vi "Main.vi"() -> ()   [LabVIEW 2017, in "Server.lvlib"]
doc: "This is the Main VI of the Dashboard Server Application. It consists of a QMH with several Loops. See the loop descriptions for details."
uses:
  Server.lvlib
  TypeDefs/SR List.ctl
  TypeDefs/SR Data.ctl
  TypeDefs/ClientList.ctl
  TypeDefs/ClientData.ctl
  SubLibs/Message Queue/EnqueueMessage(Single).vi
  <vilib>/Utility/error.llb/Error Cluster From Error Code.vi
  <vilib>/ErrorRing/Error Ring.xnode
  SubLibs/Message Queue/Message Queue.lvlib
  SubLibs/ErrorLogger/ErrorLogger.lvlib
  SubLibs/Oracle/Oracle.lvlib
  SubLibs/WebServiceCommunication/WebServiceCommunication.lvlib
  SubLibs/Logging/Logging.lvlib
  SubLibs/Timing/Timing.lvlib
  SubLibs/Dialogs/Dialogs.lvlib
panel:
  in  "LaunchSettings":bool
  in  "Tab Control":T1(tab)
  in  "RefreshSRs":bool
  in  "FilterSRs":bool
  out "SRs":string[][](table)=[["3060161", "AE-Poland", "Adriana Stepien", "Sample missing - TotalSampPerChannel results one less sample", "16.01.2018 - 09:57", "Witold", "Klopot", "Tenneco Automotive Polska Sp. z o.o. (PL)", "26.07.2017 - 05:10", "LV", "IN WORK Wait on Customer", "Standard | Active 30-Day", "PHONE", "176,2"], ["3075745", "AE-Hungary", "Daniel Fulop", "cRIO-9068 STATUS LED flashes 4 times", "10.01.2018 - 01:46", "Zsolt", "Zavori", "Vesz-Mont 2000. Kft. (HU)", "18.09.2017 - 06:08", "RIO", "IN WORK Escalation", "Premier | KEYCP, SRLLEASE", "PHONE", "122,1"], ["3083157", "AE-Poland", "Adriana Stepien", "Deploying the Mainsequence with all additional files, to the closed-code file, which can be run in customized sequencer.", "09.01.2018 - 04:42", "Konrad", "Konopka", "Woodward Inc", "13.10.2017 - 04:19", "TestStand", "IN WORK Wait on Customer", "Standard | Global VLA", "PHONE", " 97,2"], ["3084717", "AE-Poland", "Katarzyna Kaminska", "Test application in C#", "16.11.2017 - 03:26", "Marcin", "Pilch", "Kimball Electronics Poland Sp. z o.o (PL)", "19.10.2017 - 01:51", "LV", "IN WORK Wait on Customer", "Basic | No Contracts", "PHONE", " 91,3"], ["3086145", "AE-Poland", "Katarzyna Kaminska", "biblioteka NI Modbus Library", "18.01.2018 - 08:07", "Kamil", "Kos", "Woodward Inc", "24.10.2017 - 05:32", "LV", "IN WORK Wait on Customer", "Standard | Global VLA", "PHONE", " 86,2"], ["3089872", "AE-Romania", "Mihai Dornea", "Logging data at certain rates", "14.12.2017 - 03:03", "Ovidiu", "Popescu", "Sangari Engineering Services (Romania) S.R.L. (RO)", "06.11.2017 - 04:55", "LV", "IN WORK Wait on Customer", "Standard | SRLLEASE", "PHONE", " 73,2"], ["3097834", "AE-Poland", "Mateusz Loska", " Error -63044 on power up disappears after cRIO reset", "04.01.2018 - 07:55", "Slawomir", "Melech", "Infotech Przemyslowe Technologie Informatyczne i Systemy Pomiarowe (PL)", "30.11.2017 - 08:17", "LV", "IN WORK", "Standard | Active 30-Day", "PHONE", " 49,0"], ["3098805", "AE-Poland", "Adriana Stepien", "NI LabWindows?/CVI? Signal Processing Toolkit 7.0.2 - installer doesn't work on Windows 7", "09.01.2018 - 08:33", "Grzegorz", "Labecki", "Centrum Diagnostyki i Ruroc.i Aparatury sp. z.o.o. (PL)", "04.12.2017 - 07:31", "LabWindows_CVI", "IN WORK", "Basic | No Contracts", "PHONE", " 45,1"], ["3100090", "AE-Poland", "Adriana Stepien", "cDAQ 9133 no connetcion over LAN, -88900 error", "10.01.2018 - 02:30", "Wojciech", "Kubicki", "Politechnika Wroclawska (PL)", "07.12.2017 - 03:49", "MultifunctionDAQ", "IN WORK Wait on Customer", "Standard | EDU", "PHONE", " 42,2"], ["3100360", "AE-Hungary", " AE, Engineer", "error: Undefined symbol at Vision Example", "08.12.2017 - 14:41", "Forum", "Contact", "National Instruments Web Support Organization", "07.12.2017 - 19:42", "LabWindows_CVI", "Open", "Basic | No Contracts", "WEB", " 41,6"], ["3100682", "AE-Hungary", " AE, Engineer", "Best way to share one boolean between parallel loops", "08.12.2017 - 19:48", "Forum", "Contact", "National Instruments Web Support Organization", "08.12.2017 - 18:16", "LV", "Open", "Basic | No Contracts", "WEB", " 40,6"], ["3100692", "AE-Hungary", " AE, Engineer", "PXIe-5624 and PXIe-5644R bit file generation", "08.12.2017 - 22:02", "Forum", "Contact", "National Instruments Web Support Organization", "08.12.2017 - 22:02", "PXI Controllers, Chassis, MXI", "Open", "Basic | No Contracts", "WEB", " 40,5"], ["3101298", "AE-Hungary", " AE, Engineer", "256 QAM", "12.12.2017 - 21:52", "Forum", "Contact", "National Instruments Web Support Organization", "12.12.2017 - 03:35", "LV", "Open", "Basic | No Contracts", "WEB", " 37,2"], ["3101306", "AE-Poland", "Katarzyna Kaminska", "NI PXI 1065, kontrolert 8106, karta 6120, TB 2708", "18.01.2018 - 07:31", "Maciej", "Dorczuk", "Wojskowy Instytut Techniki Pancernej i Samochodowej (PL)", "12.12.2017 - 03:57", "LV", "IN WORK Wait on Customer", "Basic | No Contracts", "PHONE", " 37,2"], ["3102156", "AE-Poland", "Adriana Stepien", "sbRIO 9651", "16.01.2018 - 08:09", "Krzysztof", "Falkowski", "Wojskowa Akademia Techniczna im. Jaroslawa Dabrowskiego (PL)", "14.12.2017 - 06:24", "RIO", "IN WORK Wait on Customer", "Standard | EDU", "PHONE", " 35,1"], ["3102184", "AE-Romania", "Mihai Dornea", "NI MAX Issue", "15.01.2018 - 04:38", "Damjan", "Drozg", "National Instruments Slovenia d.o.o.   (SI)", "14.12.2017 - 08:27", "LV", "IN WORK", "Standard | SRLLEASE", "PHONE", " 35,0"], ["3102905", "AE-Hungary", "Ambrus Gregor", "Low current measurement", "17.01.2018 - 07:24", "Istvan", "Farkas", "Videoton EAS Kft. (HU)", "18.12.2017 - 03:41", "DMM", "IN WORK Wait on Customer", "Basic | No Contracts", "PHONE", " 31,2"], ["3103342", "AE-Poland", "Andrzej Filipek", "Wolno dzialajacy PXI 8115", "16.01.2018 - 03:25", "Zbigniew", "Pudlo", "WSK PZL-Swidnik SA (PL)", "19.12.2017 - 05:56", "PXI Controllers, Chassis, MXI", "IN WORK Wait on Customer", "Basic | No Contracts", "PHONE", " 30,1"], ["3104326", "AE-Hungary", " AE, Engineer", "OPC UA toolkit can't get value", "21.12.2017 - 19:17", "Forum", "Contact", "National Instruments Web Support Organization", "21.12.2017 - 19:17", "LV", "Open", "Basic | No Contracts", "WEB", " 27,6"], ["3105279", "AE-Hungary", " AE, Engineer", "LabVIEW and communication via Profinet", "28.12.2017 - 20:22", "Forum", "Contact", "National Instruments Web Support Organization", "28.12.2017 - 20:22", "LV", "Open", "Basic | No Contracts", "WEB", " 20,5"], ["3106913", "AE-Poland", "Adriana Stepien", "How to change data between FPGA and Host", "11.01.2018 - 02:11", "Wojciech", "Krawczyk", "ABIS SP Z O O SPOLKA KOMANDYTOWA (PL)", "08.01.2018 - 07:12", "LVFPGA", "IN WORK", "Basic | No Contracts", "PHONE", " 10,1"], ["3107367", "AE-Czech Republic", "Michal Jadrny", "Using 100kHz/Timebase signal as a clock signal for Finite Input measurement", "18.01.2018 - 09:00", "Lubomir", "Losonsky", "KOSTAL CR Spol. s r.o. (CZ)", "09.01.2018 - 08:56", "MStudioDotNet", "IN WORK", "Premier | KEYCP", "PHONE", "  9,0"], ["3108038", "AE-Hungary", " AE, Engineer", "LV text rendering, MBCS, OS, Unicode", "17.01.2018 - 21:16", "Forum", "Contact", "National Instruments Web Support Organization", "11.01.2018 - 01:29", "LV", "Open", "Basic | No Contracts", "WEB", "  7,3"], ["3108128", "AE-Hungary", "Ambrus Gregor", "Decimal representation conflict", "17.01.2018 - 03:56", "Gergo", "Vajas", "Cobra Control Kft.(HU)", "11.01.2018 - 05:33", "LV", "IN WORK Wait on Customer", "Standard | SRLLEASE", "PHONE", "  7,2"], ["3108306", "AE-Hungary", " AE, Engineer", "*** How to generate a function panel file (.fp) properly in CVI ***", "12.01.2018 - 14:55", "Forum", "Contact", "National Instruments Web Support Organization", "11.01.2018 - 14:41", "LabWindows_CVI", "Open", "Basic | No Contracts", "WEB", "  6,8"], ["3108584", "AE-Hungary", "Ambrus Gregor", "Loging in to database with different names", "17.01.2018 - 03:56", "Damjan", "Remih", "Danfoss Trata d.o.o.      (SI)", "12.01.2018 - 08:04", "TestStand", "IN WORK Wait on Customer", "Basic | No Contracts", "PHONE", "  6,0"], ["3108586", "AE-Poland", "Adriana Stepien", "Merging two projects into one", "16.01.2018 - 03:37", "Mariusz", "Wicinski", "K & M SoftControl  (DE)", "12.01.2018 - 08:12", "LV", "IN WORK Wait on Customer", "Standard | SSP", "PHONE", "  6,0"], ["3108737", "AE-Hungary", " AE, Engineer", "LabVIEW RTE patch version mismatch and adapter error", "16.01.2018 - 23:21", "Forum", "Contact", "National Instruments Web Support Organization", "12.01.2018 - 20:35", "TestStand", "Open", "Basic | No Contracts", "WEB", "  5,5"], ["3108874", "AE-Czech Republic", "Patrik Karandusovsky", "FPGA modul pro Windows 10", "18.01.2018 - 03:24", "Zdenek", "Mastnik", "Zdenek Mastnik Vyvoj SW a HW (CZ)", "15.01.2018 - 01:19", "LV", "IN WORK Wait on Customer", "Standard | SRLLEASE", "PHONE", "  3,3"], ["3108882", "AE-Czech Republic", "Michal Jadrny", "kompilace kodu", "16.01.2018 - 09:39", "Karel", "Svajda", "Karel Svajda (CZ)", "15.01.2018 - 01:39", "LV", "IN WORK", "Standard | SSP", "PHONE", "  3,3"], ["3108931", "AE-Hungary", " AE, Engineer", "Configuration Problem with LV 2010", "15.01.2018 - 04:09", "Tamas", "Makk", "BPW Hungaria Kft  (HU)", "15.01.2018 - 04:06", "LV", "Open", "Standard | Active 30-Day", "PHONE", "  3,2"], ["3108950", "AE-Hungary", "Tamas Virag", "Unable to converge during transient analysis", "17.01.2018 - 08:57", "Peter", "Severnyak", "Vincotech Hungaria Kft.  (HU)", "15.01.2018 - 05:10", "Multisim (EWB)", "IN WORK", "Standard | SSP", "PHONE", "  3,2"], ["3108973", "AE-Romania", "Denis Stavila", "How many DRAM memory item data can I define without overloading DRAM Arbiter", "16.01.2018 - 04:27", "Vuk", "Obradovic", "Forsteh d.o.o. (SI)", "15.01.2018 - 07:29", "LVFPGA", "IN WORK", "Standard | SRLLEASE", "PHONE", "  3,1"], ["3108982", "AE-Hungary", "Tamas Virag", "Acces to LV 2013 SP1", "18.01.2018 - 08:37", "Lorant", "Szasz", "Robert Bosch Energy & Body Systems Kft.  (HU)", "15.01.2018 - 07:48", "LV", "IN WORK", "Basic | No Contracts", "PHONE", "  3,0"], ["3109029", "AE-Poland", "Katarzyna Kaminska", "(p) szybkosc przeladowania interfaceow, LabView", "18.01.2018 - 07:27", "Agnieszka", "Lisicka", "Fitech Sp. z o.o. (PL)", "15.01.2018 - 09:46", "LV", "IN WORK Wait on Customer", "Standard | Global VLA, SRLLEASE", "PHONE", "  3,0"], ["3109167", "AE-Hungary", " AE, Engineer", "Reading, writing and sending http request using myRio", "15.01.2018 - 19:11", "Forum", "Contact", "National Instruments Web Support Organization", "15.01.2018 - 19:11", "MultifunctionDAQ", "Open", "Basic | No Contracts", "WEB", "  2,6"], ["3109321", "AE-Hungary", "Ambrus Gregor", "What is the compatibility between the DAQmx LabVIEW and TestStand versions?", "18.01.2018 - 03:31", "Zoltan", "Vanyi", "ENG Systems Hungary Kft  (HU)", "16.01.2018 - 04:01", "LV", "IN WORK Wait on Customer", "Standard | SRLLEASE", "PHONE", "  2,2"], ["3109336", "AE-Romania", "Mihai Dornea", "[LOC][PHONE] - M83X09560", "18.01.2018 - 08:32", "Arnaud", "Dumont", "teamtechnik Maschinen und Anlagen GmbH  (DE)", "16.01.2018 - 04:41", "LV", "Open", "Standard | Active 30-Day", "PHONE", "  2,2"], ["3109341", "AE-Czech Republic", " AE, Engineer", "Traceable calibration for NI PXI-4065", "16.01.2018 - 05:05", "David", "Svikruha", "ALPHA Vehicle Security Solutions Czech s.r.o. (CZ)", "16.01.2018 - 05:05", "LV", "Open", "Basic | No Contracts", "PHONE", "  2,2"], ["3109357", "AE-Romania", "Mihai Dornea", "NI-9860 faulty", "17.01.2018 - 06:56", "Marius", "Galatan", "Continental Automotive Systems S.R.L (RO)", "16.01.2018 - 06:43", "CM C Series", "IN WORK Wait on Customer", "Standard | Global VLA", "PHONE", "  2,1"], ["3109623", "AE-Hungary", " AE, Engineer", "3D picture controll + CTRL + SHIFT keys", "17.01.2018 - 01:11", "Forum", "Contact", "National Instruments Web Support Organization", "16.01.2018 - 21:28", "LV", "Open", "Basic | No Contracts", "WEB", "  1,5"], ["3109684", "AE-Poland", "Adriana Stepien", "Technische Fragen bzgl. Verbindung mit dem OPC Server (LV 2015)", "17.01.2018 - 04:45", "Friedrich", "Seidel", "Leonhard Kurz Stiftung & Co.KG (DE)", "17.01.2018 - 01:18", "OPC Servers", "IN WORK", "Standard | SSP", "PHONE", "  1,3"], ["3109723", "AE-Romania", "Mihai Dornea", "Provide a temporary license for VBAI", "17.01.2018 - 02:49", "Bogdan", "Balauta", "National Instruments Romania (RO)", "17.01.2018 - 02:45", "VisionSW", "IN WORK Wait on Customer", "Basic | No Contracts", "PHONE", "  1,3"], ["3109727", "AE-Poland", "Andrzej Filipek", "Problem z pobraniem LabVIEW", "18.01.2018 - 05:46", "Andrzej", "Jaeschke", "Politechnika Lodzka (PL)", "17.01.2018 - 02:55", "LV", "IN WORK Wait on Customer", "Basic | No Contracts", "PHONE", "  1,3"], ["3109816", "AE-Czech Republic", "Michal Jadrny", "Trobleshooting for driver for Labview", "18.01.2018 - 02:05", "Jindrich", "Fiala", "T-Mobile Czech Republic a.s. (CZ)", "17.01.2018 - 07:50", "LV", "IN WORK", "Standard | SRLLEASE", "PHONE", "  1,1"], ["3110007", "AE-Hungary", " AE, Engineer", "Help with identification of CLD-like problem", "18.01.2018 - 00:48", "Forum", "Contact", "National Instruments Web Support Organization", "17.01.2018 - 20:11", "LV", "Open", "Basic | No Contracts", "WEB", "  0,5"], ["3110158", "AE-Hungary", " AE, Engineer", "memristor simulation", "18.01.2018 - 05:03", "Forum", "Contact", "National Instruments Web Support Organization", "18.01.2018 - 05:03", "Multisim (EWB)", "Open", "Basic | No Contracts", "WEB", "  0,2"], ["3110178", "AE-Romania", "Mihai Dornea", "clearing tasks in MAX", "18.01.2018 - 07:25", "Gheorghe", "Dragan", "Gheorghe Dragan (RO)", "18.01.2018 - 06:55", "MultifunctionDAQ", "IN WORK", "Basic | No Contracts", "PHONE", "  0,1"], ["3110193", "AE-Czech Republic", "Michal Jadrny", "Problem with detecting cDAQ-9185", "18.01.2018 - 08:01", "Frantisek", "Vrba", "Continental Automotive Czech Republic s.r.o. (CZ)", "18.01.2018 - 07:50", "MultifunctionDAQ", "IN WORK", "Standard | SSP", "PHONE", "  0,1"], ["3110195", "AE-Poland", "Katarzyna Kaminska", "Detailed specification question about NI 9205", "18.01.2018 - 07:55", "Lukasz", "Przystalski", "PBP Enamor Sp. z o.o.  (PL)", "18.01.2018 - 07:54", "MultifunctionDAQ", "IN WORK", "Basic | No Contracts", "PHONE", "  0,1"], ["3110202", "AE-Czech Republic", " AE, Engineer", "Trobleshooting for measuring in NI DAQ", "18.01.2018 - 08:46", "Martin", "Kralik", "Ceske vysoke uceni technicke v Praze (CZ)", "18.01.2018 - 08:10", "LV", "Open", "Standard | EDU", "PHONE", "  0,0"], ["3110207", "AE-Hungary", "Tamas Virag", "Pinout for NI9421 for encoder", "18.01.2018 - 08:32", "Marton", "Litkei", "National Instruments Hungary Kft (HU)", "18.01.2018 - 08:29", "RIO", "IN WORK", "Standard | SRLLEASE", "PHONE", "  0,0"], ["3110215", "AE-Hungary", "Tamas Virag", "DAQmxGetDeviceAttribute on NI-4082", "18.01.2018 - 08:59", "Zsolt", "Horvath", "Robert Bosch Kft. (HU)", "18.01.2018 - 08:43", "DMM", "IN WORK", "Standard | Global VLA", "PHONE", "  0,0"], ["7705656", "AE-Poland", "Mateusz Loska", "calling .net assemblies created from labview somethimes hangs powershell", "02.08.2017 - 06:28", "Tobiasz", "Heller", "Politechnika Slaska (PL)", "30.03.2017 - 04:56", "LV", "IN WORK Customer Added Note", "Standard | Global VLA, EDU", "EMAIL", "294,2"], ["7711599", "AE-Romania", "Mihai Dornea", "Database toolkit reconnect", "11.01.2018 - 06:01", "Martin", "Kas", "Zapadoceska univerzita v Plzni   (CZ)", "21.06.2017 - 04:04", "LV", "IN WORK Wait on Customer", "Standard | EDU", "EMAIL", "211,2"], ["7723886", "AE-Czech Republic", "Michal Jadrny", "LV app performance problems on server with dual XEON E5-2630 (Win. Server 2012)", "16.01.2018 - 09:39", "Petr", "Preucil", "T-Mobile Czech Republic a.s. (CZ)", "07.11.2017 - 09:25", "LV", "IN WORK", "Standard | SRLLEASE", "PHONE", " 72,0"], ["7725759", "AE-Czech Republic", "Patrik Karandusovsky", "3D picture VRL model overlaping", "15.01.2018 - 02:56", "Pawel", "Hanus", "Hanus Pawel (PL)", "28.11.2017 - 08:41", "LV", "IN WORK Escalation", "Basic | No Contracts", "EMAIL", " 51,0"], ["7726610", "AE-Hungary", "Ambrus Gregor", "NI Application Web Server hanging", "18.01.2018 - 03:19", "Lukas", "Hostalek", "ATS aplikovane technicke systemy s.r.o.  (CZ)", "07.12.2017 - 01:41", "LV", "IN WORK Escalation", "Standard | SRLLEASE", "EMAIL", " 42,3"], ["7726642", "AE-Romania", "Denis Stavila", "A dinamic link library (DLL) initialization routine failed", "09.01.2018 - 02:15", "Cenusa", "Daniel", "Continental Automotive Romania SRL (RO)", "07.12.2017 - 08:48", "LV", "IN WORK Customer Added Note", "Standard | Global VLA, SSP", "EMAIL", " 42,0"], ["7727096", "AE-Poland", "Adriana Stepien", "Problem z komunikacja szeregowa przez port USB (uklad FTDI, PORT COM)", "08.01.2018 - 04:32", "Michal", "Mirowski", "TRW Polska Sp.z o.o (PL)", "13.12.2017 - 01:47", "LV", "IN WORK Wait on Customer", "Standard | Special VLA", "PHONE", " 36,3"], ["7727100", "AE-Poland", "Mateusz Loska", "Designing user specified RMC", "02.01.2018 - 03:38", "Przemyslaw", "Bibik", "Politechnika Warszawska (PL)", "13.12.2017 - 02:11", "LV", "IN WORK", "Standard | EDU", "EMAIL", " 36,3"], ["7728306", "AE-Slovakia", "Michal Jadrny", "Offline licenses not working as expected (M76X36531)", "11.01.2018 - 07:41", "Juraj", "Talan", "Kistler Bratislava, s.r.o. (SK)", "04.01.2018 - 01:45", "LV", "IN WORK Escalation", "Standard | SSP", "EMAIL", " 14,3"], ["7728804", "AE-Poland", "Adriana Stepien", "NI9882 - EDS revision error", "18.01.2018 - 08:12", "Adrian", "Krol", "General Motors Manufacturing Poland Sp. z o.o. (PL)", "10.01.2018 - 03:54", "Industrial Communications", "IN WORK Wait on Customer", "Standard | Global VLA", "EMAIL", "  8,2"], ["7729076", "AE-Hungary", "Ambrus Gregor", "Access is denied Error - 17205", "18.01.2018 - 07:06", "Marko", "Plenkovic", "RT-RK Institute for Computer Based Systems (SI)", "12.01.2018 - 05:14", "TestStand", "IN WORK Wait on Customer", "Basic | No Contracts", "EMAIL", "  6,2"], ["7729172", "AE-Hungary", "Ambrus Gregor", "LDAP support and configuration in NI Volume License Manager", "17.01.2018 - 03:56", "Asdrubal", "Mendes", "Melexis Bulgaria Ltd. (SI)", "14.01.2018 - 16:10", "VolumeLicenseMgr", "IN WORK Wait on Customer", "Standard | Global VLA", "EMAIL", "  3,7"], ["7729217", "AE-Hungary", "Ambrus Gregor", "LV2015 - DSC runtime - Win10 update Issue", "18.01.2018 - 08:44", "Damir", "Krovinovic", "Krovel d.o.o. (SI)", "15.01.2018 - 07:02", "LV", "IN WORK Wait on Customer", "Basic | No Contracts", "EMAIL", "  3,1"], ["7729319", "AE-Czech Republic", "Michal Jadrny", "nastaveni vysoke samplovani pouze na jedne karte ( 10kHz) a nizke freq P loop", "17.01.2018 - 08:32", "Vaclav", "Rychtar", "Skoda Auto a.s. (CZ)", "16.01.2018 - 04:29", "VeriStand", "IN WORK", "Standard | Global VLA, SSP", "PHONE", "  2,2"], ["7729339", "AE-Poland", " AE, Engineer", "Teststand code source control with subversion", "16.01.2018 - 08:13", "Lukasz", "Kwiatkowski", "Politechnika Slaska (PL)", "16.01.2018 - 08:13", "LV", "Open", "Premier | VAR+, EDU", "EMAIL", "  2,0"]]
  out "Last Update SRs":timestamp
  in  "Launch Event Log":bool
  in  "Launch Export":bool
  in  "Launch Statistics":bool
  in  "LaunchTestClient":bool
  out "Last Update Clients":timestamp
  in  "GetCurrentClients":bool
  out "Clients":string[][](table)
  in  "Exit":bool
  # "CER AE DASHBOARD SERVER"
  # "We could implement a subpanel here instead of the dialog-popups"
  # "Have your commercials here"
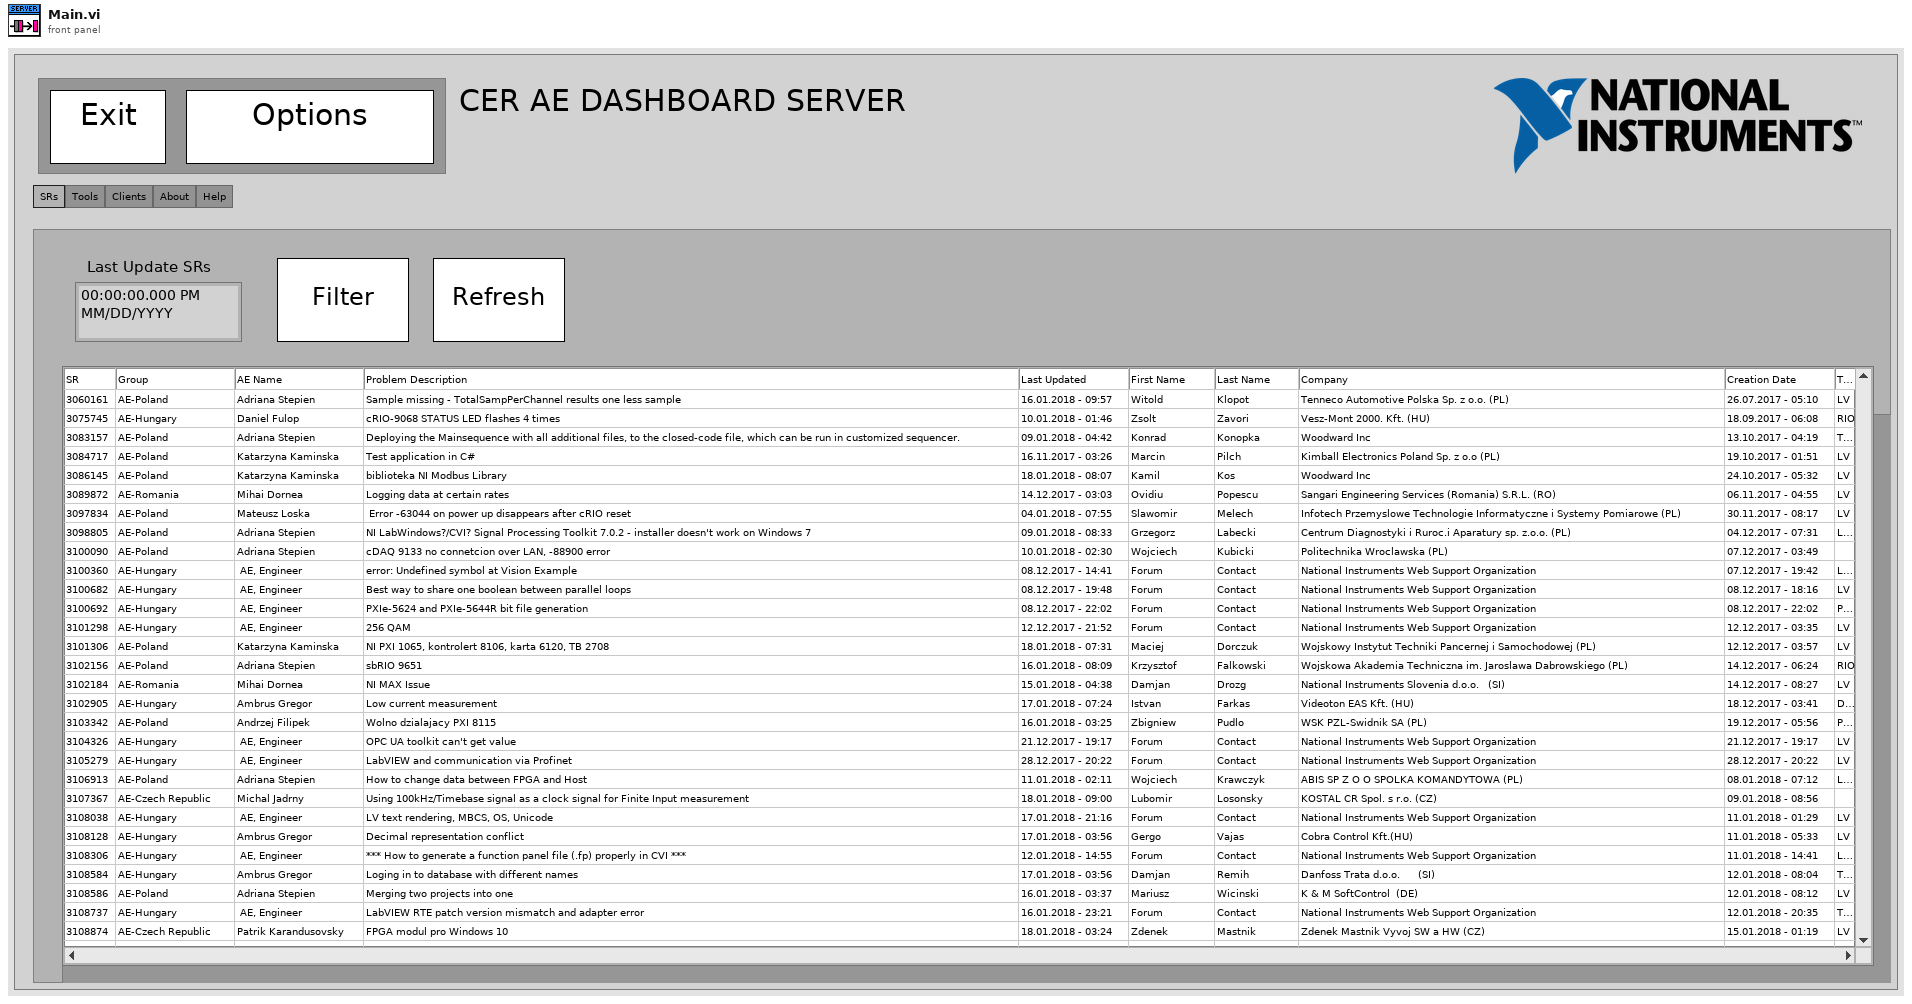
[diagram p1: front panel]
types:
  T1 = enum32{"SRs", "Tools", "Clients", "About", "Help"}
  T2 = typedef "Server.lvlib/Message Queue.lvlib/CommReferences.ctl" = cluster{"MHL":refnum<queue>, "Error":refnum<queue>, "EventReg":refnum<event-registration>, "Event":refnum<user-event>, "UI":refnum<queue>, "WebServ":refnum<queue>, "Oracle":refnum<queue>, "Timing":refnum<queue>, "Log":refnum<queue>, "Dialog":refnum<queue>}
  T3 = typedef "Server.lvlib/SR List.ctl" = T4[]
  T4 = typedef "Server.lvlib/SR Data.ctl" = cluster{"SR#":dbl, "Group":string, "Owner":string, "Problem Summary":string, "Last Updated":timestamp, "Customer First Name":string, "Customer Last Name":string, "Company":string, "Created On":timestamp, "SR Type":string, "Status":string, "Service Level":string, "Channel":string, "Days Open":dbl}
  T5 = typedef "Server.lvlib/ClientList.ctl" = T6[]
  T6 = typedef "Server.lvlib/ClientData.ctl" = cluster{"ClientID":string, "LastHeartbeat":timestamp}
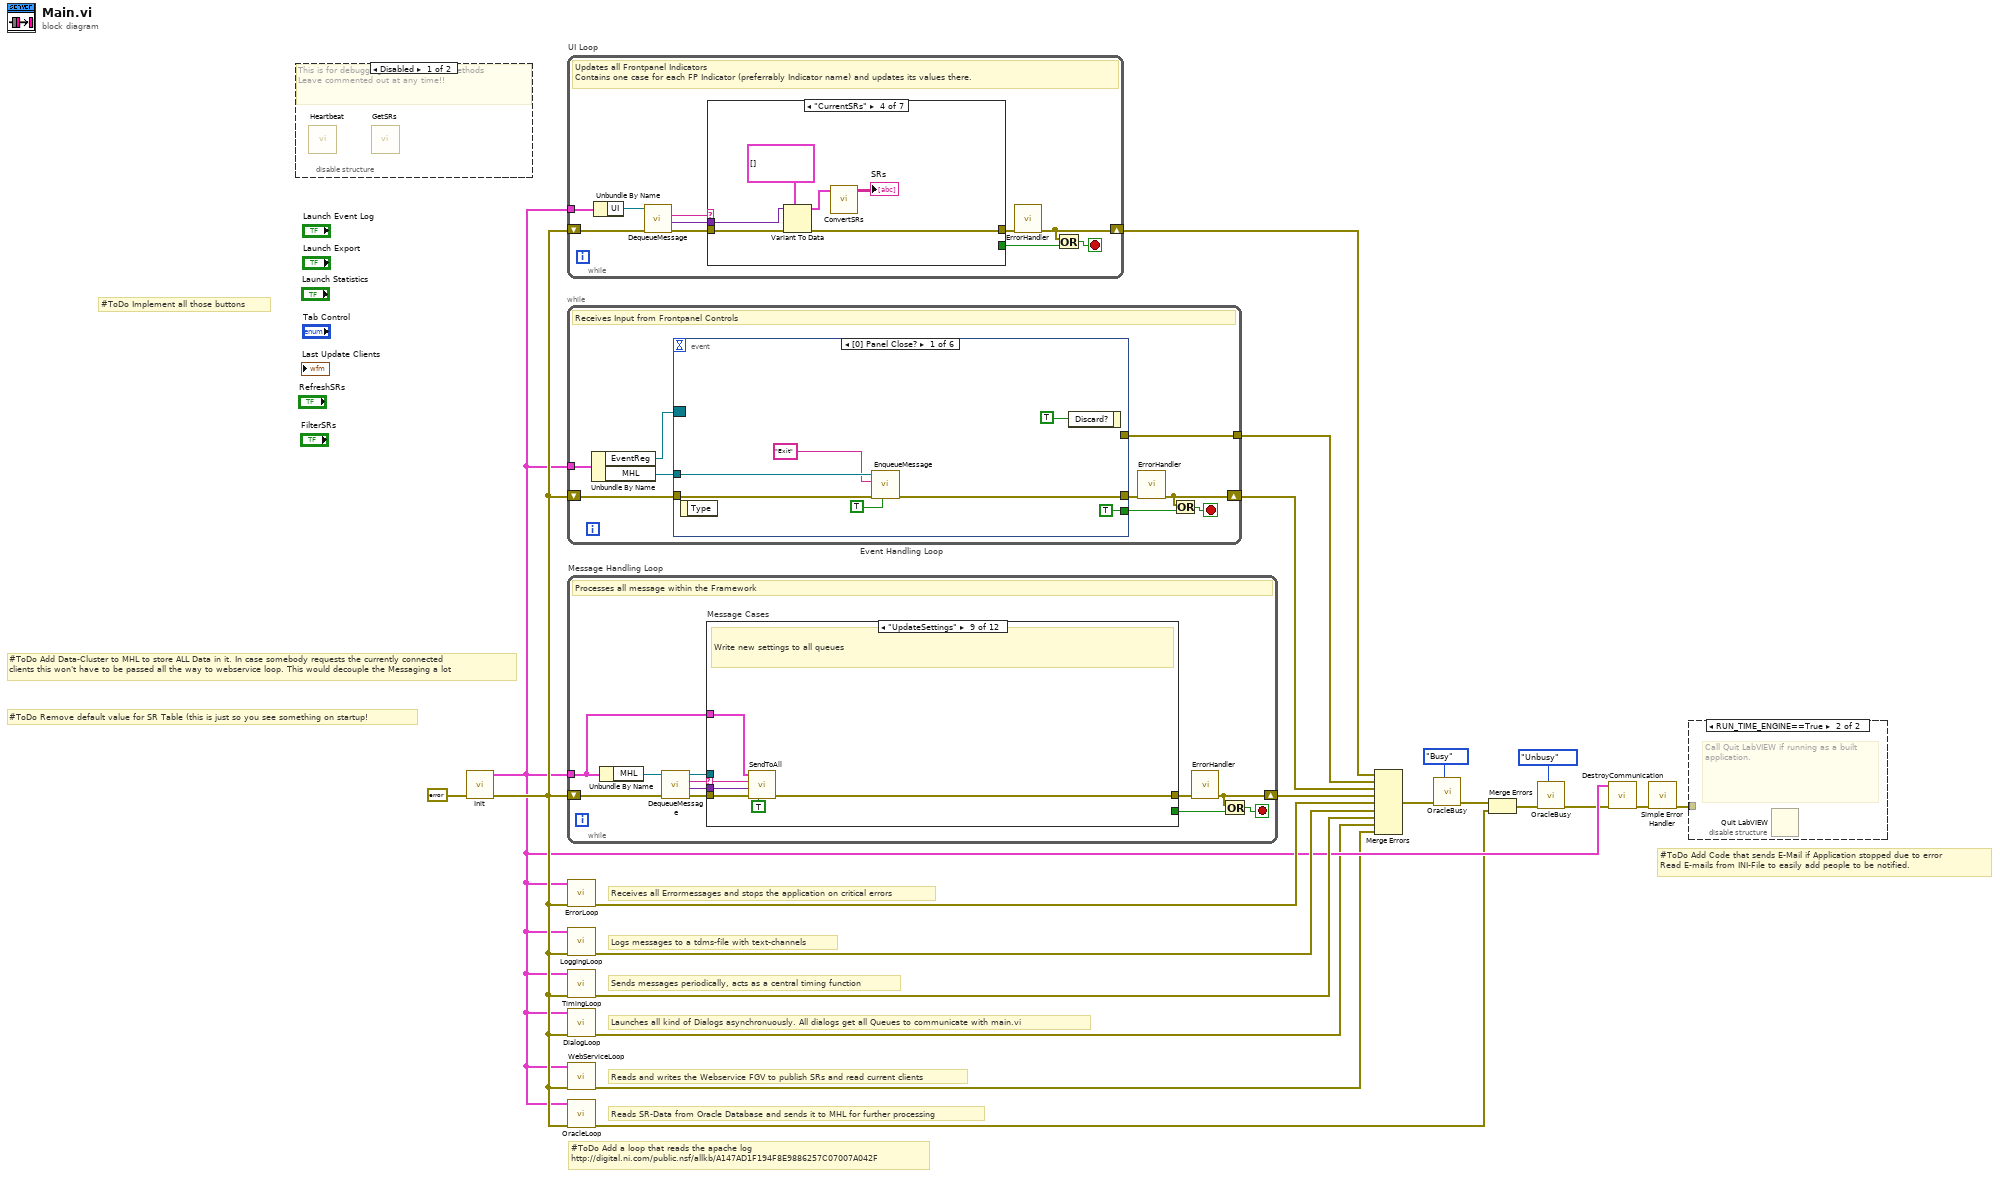
[diagram p0: block diagram]
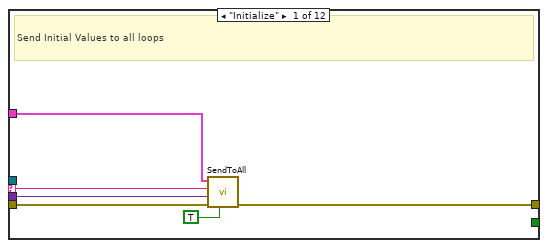
[diagram p2: hidden frame]
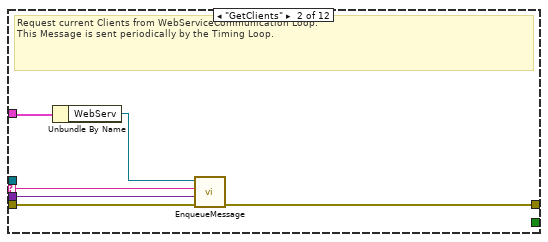
[diagram p3: hidden frame]
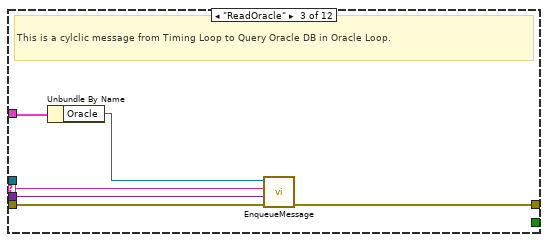
[diagram p4: hidden frame]
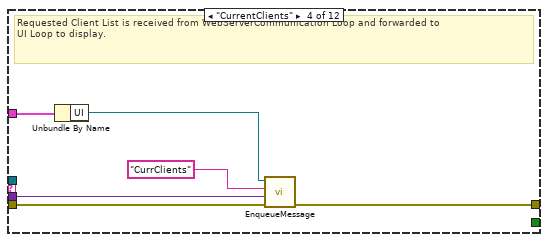
[diagram p5: hidden frame]
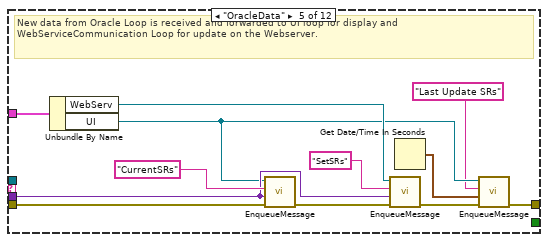
[diagram p6: hidden frame]
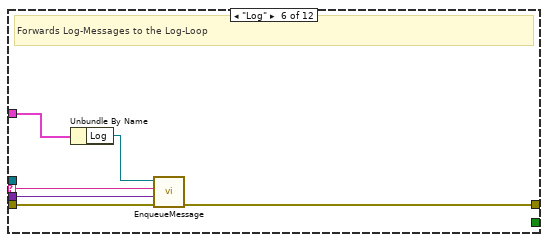
[diagram p7: hidden frame]
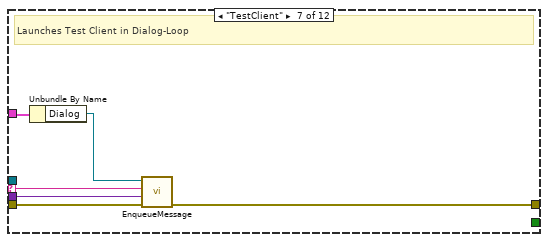
[diagram p8: hidden frame]
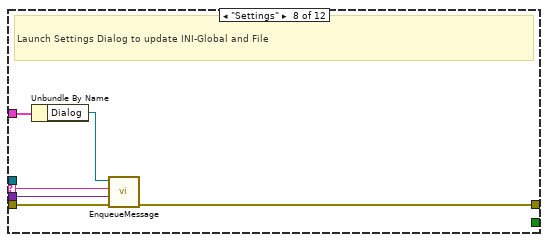
[diagram p9: hidden frame]
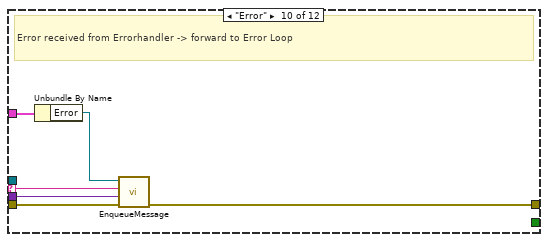
[diagram p10: hidden frame]
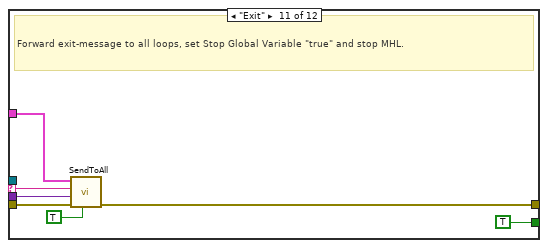
[diagram p11: hidden frame]
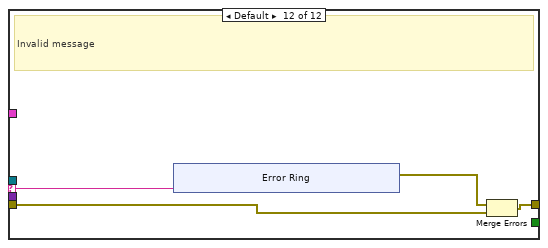
[diagram p12: hidden frame]
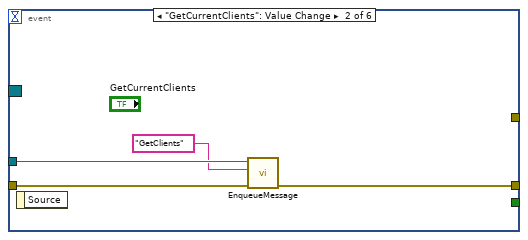
[diagram p13: hidden frame]
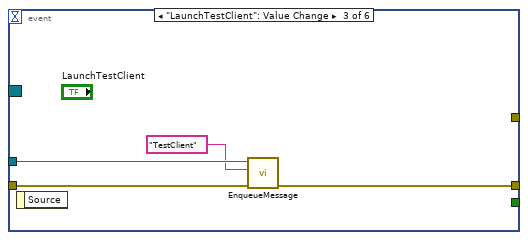
[diagram p14: hidden frame]
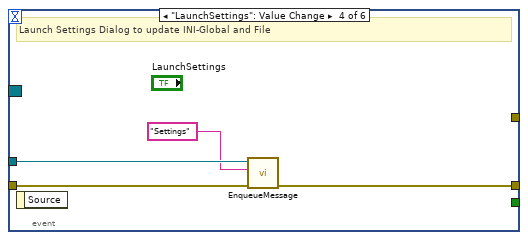
[diagram p15: hidden frame]
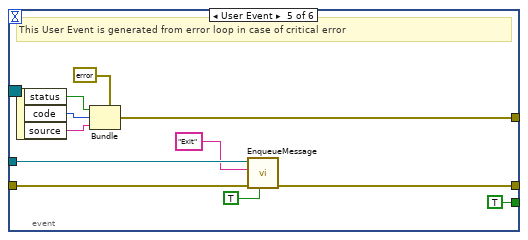
[diagram p16: hidden frame]
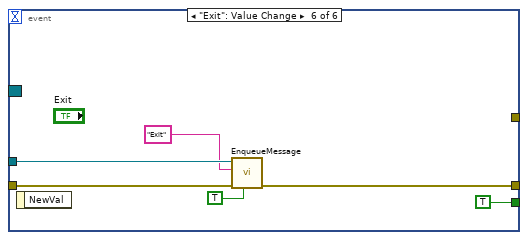
[diagram p17: hidden frame]
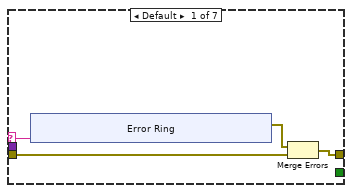
[diagram p19: hidden frame]
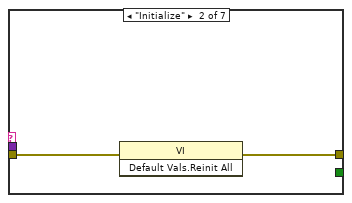
[diagram p20: hidden frame]
diagram:
  # "#ToDo Implement all those buttons"
  # "#ToDo Remove default value for SR Table (this is just so you see something on startup!"
  # "#ToDo Add Data-Cluster to MHL to store ALL Data in it. In case somebody requests the currently connected\nclients this won't have to be passed all the way to webservice loop. This would decouple the Messaging a lot"
  # "Launches all kind of Dialogs asynchronuously. All dialogs get all Queues to communicate with main.vi"
  # "Reads and writes the Webservice FGV to publish SRs and read current clients"
  # "Reads SR-Data from Oracle Database and sends it to MHL for further processing"
  # "Sends messages periodically, acts as a central timing function"
  # "Logs messages to a tdms-file with text-channels"
  # "Receives all Errormessages and stops the application on critical errors"
  # "#ToDo Add Code that sends E-Mail if Application stopped due to error\nRead E-mails from INI-File to easily add people to be notified."
  # "#ToDo Add a loop that reads the apache log\nhttp://digital.ni.com/public.nsf/allkb/A147AD1F194F8E9886257C07007A042F"
  n1 = disable-structure shown="Disabled" {
    frame Disabled {
      # "This is for debugging the Webservice Methods\nLeave commented out at any time!!"
      n2 = call "Heartbeat.vi"() -> ()  [unwired: 12 in]
      n3 = call "GetSRs.vi"() -> ()  [unwired: 11 in, 1 out]
    }
    frame Enabled {
    }
  }
  n4 = call "Init.vi"("error in (no error)"=errorcluster {"status"=FALSE, "code"=0, "source"=""}) -> ("error out"=w12:errorcluster, "Message Queues out"=w11:T2)  [unwired: 9 in]
  n5 = while "UI Loop" {
    shift-right: [w22] -> w15
    shift-left: w12 -> [w31]
    tunnel: w11 -> [w30]
    stop <- w23 stop-if-true
    # "Updates all Frontpanel Indicators\nContains one case for each FP Indicator (preferrably Indicator name) and updates its values there."
    n6 = Unbundle By Name(w30) -> ("UI"=w29:refnum<queue>)
    n7 = call "DequeueMessage.vi"("error in (no error)"=w31, "Message Queue"=w29) -> ("error out"=w27:errorcluster, "Message Data"=w25:variant, "Message"=w28:string)  [unwired: 5 in, 2 out]
    n8 = case shown="\"CurrentSRs\"" w28 {
      selector: w28 -> [w34 _ _ _ _ _ _]
      tunnel: [w33 w43 w45 w50 w56 w61 w64] -> w26
      tunnel: w27 -> [w35 w44 w45 w51 w57 w62 w64]
      tunnel: w25 -> [_ _ _ w48 w55 w60 _]
      tunnel: [_ _ _ _ _ _ TRUE] -> w24
      frame Default {
        n9 = xnode "Error Ring"("parameter 0"=w34) -> ("error out"=w32:errorcluster)
        n10 = Merge Errors(w32, w35) -> (w33:errorcluster)
      }
      frame "Initialize" {
        n11 = invoke class="VI" method="Default Vals.Reinit All"(error in=w44) -> (error out=w43:errorcluster)  [unwired: 2 in, 2 out]
      }
      frame "UpdateSettings" {
        # "Updates any Values from INI, not used yet"
      }
      frame "CurrentSRs" {
        n12 = Variant To Data(error in=w51, type=T3 [] ("CurrentSRs"), Variant=w48) -> (data=w47:T3, error out=w50:errorcluster)
        n13 = call "ConvertSRs.vi"("SRList"=w47) -> ("SRlistString"=→"SRs":string[][])  [unwired: 10 in]
      }
      frame "CurrClients" {
        n14 = Variant To Data(error in=w57, type=T5 [] ("ClientList"), Variant=w55) -> (data=w53:T5, error out=w56:errorcluster)
        n15 = call "ConvertClients.vi"("ClientList"=w53) -> ("ClientListArray"=→"Clients":string[][])  [unwired: 10 in]
      }
      frame "Last Update SRs" {
        n16 = Variant To Data(error in=w62, type=timestamp(0 s since 1904-01-01) ("Time Stamp"), Variant=w60) -> (data=→"Last Update SRs":timestamp, error out=w61:errorcluster)
      }
      frame "Exit" {
      }
    }
    n17 = call "ErrorHandler.vi"("error in (no error)"=w26) -> ("error out"=w22:errorcluster)  [unwired: 10 in]
    n18 = Or(x=w22, y=w24) -> (x .or. y?=w23:bool)
  }
  n19 = while "Event Handling Loop" {
    tunnel: w11 -> [w73]
    shift-right: [w65] -> w20
    shift-left: w12 -> [w70]
    tunnel: [w68] -> w18
    stop <- w66 stop-if-true
    # "Receives Input from Frontpanel Controls"
    n20 = Unbundle By Name(w73) -> ("EventReg"=w71:refnum<event-registration>, "MHL"=w72:refnum<queue>)
    n21 = event shown="[0] Panel Close?" {
      selector: w71 -> [_ _ _ _ _ _]
      dyn-events: _ -> [_ _ _ _ _ _]
      timeout: _ -> [_ _ _ _ _ _]
      tunnel: w72 -> [w79 w82 w86 w90 w96 w109]
      tunnel: [w78 w83 w87 w91 w97 w108] -> w69
      tunnel: w70 -> [w75 w84 w88 w92 w103 w104]
      tunnel: [_ _ _ _ w98 _] -> w68
      tunnel: [TRUE ("Priority Message? (F)") _ _ _ TRUE ("Priority Message? (F)") TRUE ("Priority Message? (F)")] -> w67
      event Panel Close? {
        n22 = event-data() -> ()  [unwired: 1 in, 1 out]
        n23 = call-poly "EnqueueMessage.vi"("Priority Message? (F)"=TRUE, "error in (no error)"=w75, "Message"="Exit", "Message Queue"=w79) -> ("error out"=w78:errorcluster)  [unwired: 6 in, 1 out]
        n24 = event-data("Discard?"=TRUE) -> ()  [unwired: 1 in, 1 out]
      }
      event "GetCurrentClients": Value Change {
        n25 = event-data() -> ()  [unwired: 1 in, 1 out]
        n26 = call-poly "EnqueueMessage.vi"("error in (no error)"=w84, "Message"="GetClients", "Message Queue"=w82) -> ("error out"=w83:errorcluster)  [unwired: 7 in, 1 out]
      }
      event "LaunchTestClient": Value Change {
        n27 = event-data() -> ()  [unwired: 1 in, 1 out]
        n28 = call-poly "EnqueueMessage.vi"("error in (no error)"=w88, "Message"="TestClient", "Message Queue"=w86) -> ("error out"=w87:errorcluster)  [unwired: 7 in, 1 out]
      }
      event "LaunchSettings": Value Change {
        # "Launch Settings Dialog to update INI-Global and File"
        n29 = event-data() -> ()  [unwired: 1 in, 1 out]
        n30 = call-poly "EnqueueMessage.vi"("error in (no error)"=w92, "Message"="Settings", "Message Queue"=w90) -> ("error out"=w91:errorcluster)  [unwired: 7 in, 1 out]
      }
      event User Event {
        # "This User Event is generated from error loop in case of critical error"
        n31 = event-data() -> ("status"=w101:bool, "code"=w100:i32, "source"=w99:string)  [unwired: 1 in]
        n32 = Bundle(cluster=errorcluster {"status"=FALSE, "code"=0, "source"=""} ("error constant"), "status"=w101, "code"=w100, "source"=w99) -> (w98:errorcluster)
        n33 = call-poly "EnqueueMessage.vi"("Priority Message? (F)"=TRUE, "error in (no error)"=w103, "Message"="Exit", "Message Queue"=w96) -> ("error out"=w97:errorcluster)  [unwired: 6 in, 1 out]
      }
      event "Exit": Value Change {
        n34 = event-data() -> ()  [unwired: 1 in, 1 out]
        n35 = call-poly "EnqueueMessage.vi"("Priority Message? (F)"=TRUE, "error in (no error)"=w104, "Message"="Exit", "Message Queue"=w109) -> ("error out"=w108:errorcluster)  [unwired: 6 in, 1 out]
      }
    }
    n36 = call "ErrorHandler.vi"("error in (no error)"=w69) -> ("error out"=w65:errorcluster)  [unwired: 10 in]
    n37 = Or(x=w65, y=w67) -> (x .or. y?=w66:bool)
  }
  n38 = while "Message Handling Loop" {
    tunnel: w11 -> [w112]
    shift-right: [w110] -> w21
    shift-left: w12 -> [w119]
    stop <- w111 stop-if-true
    # "Processes all message within the Framework"
    n39 = Unbundle By Name(w112) -> ("MHL"=w114:refnum<queue>)
    n40 = call "DequeueMessage.vi"("error in (no error)"=w119, "Message Queue"=w114) -> ("error out"=w118:errorcluster, "Message Data"=w116:variant, "Message"=w117:string, "dup Message Queue"=w115:refnum<queue>)  [unwired: 5 in, 1 out]
    n41 = case "Message Cases" shown="\"UpdateSettings\"" w117 {
      selector: w117 -> [w124 w131 w134 _ _ w160 w166 w170 w177 w182 w189 w196]
      tunnel: w115 -> [_ _ _ _ _ _ _ _ _ _ _ _]
      tunnel: w118 -> [w126 w132 w138 w144 w156 w162 w168 w174 w180 w186 w192 w194]
      tunnel: [w125 w127 w137 w143 w150 w161 w167 w173 w179 w185 w190 w195] -> w113
      tunnel: [_ _ _ _ _ _ _ _ _ _ TRUE _] -> w120
      tunnel: w116 -> [w121 w130 w133 w142 w154 w159 w165 w169 w176 w181 w187 _]
      tunnel: w112 -> [w123 w129 w136 w140 w152 w158 w164 w172 w178 w184 w191 _]
      frame "Initialize" {
        # "Send Initial Values to all loops"
        n42 = call "SendToAll.vi"("Priority Message? (F)"=TRUE, "error in (no error)"=w126, "Data"=w121, "Message"=w124, "Message Queues in"=w123) -> ("error out"=w125:errorcluster)  [unwired: 6 in]
      }
      frame "GetClients" {
        # "Request current Clients from WebServiceCommunication Loop.\nThis Message is sent periodically by the Timing Loop."
        n43 = Unbundle By Name(w129) -> ("WebServ"=w128:refnum<queue>)
        n44 = call-poly "EnqueueMessage.vi"("error in (no error)"=w132, "Message Data"=w130, "Message"=w131, "Message Queue"=w128) -> ("error out"=w127:errorcluster)  [unwired: 6 in, 1 out]
      }
      frame "ReadOracle" {
        # "This is a cylclic message from Timing Loop to Query Oracle DB in Oracle Loop."
        n45 = Unbundle By Name(w136) -> ("Oracle"=w135:refnum<queue>)
        n46 = call-poly "EnqueueMessage.vi"("error in (no error)"=w138, "Message Data"=w133, "Message"=w134, "Message Queue"=w135) -> ("error out"=w137:errorcluster)  [unwired: 6 in, 1 out]
      }
      frame "CurrentClients" {
        # "Requested Client List is received from WebServerCommunication Loop and forwarded to \nUI Loop to display."
        n47 = Unbundle By Name(w140) -> ("UI"=w139:refnum<queue>)
        n48 = call-poly "EnqueueMessage.vi"("error in (no error)"=w144, "Message Data"=w142, "Message"="CurrClients", "Message Queue"=w139) -> ("error out"=w143:errorcluster)  [unwired: 6 in, 1 out]
      }
      frame "OracleData" {
        # "New data from Oracle Loop is received and forwarded to UI loop for display and WebServiceCommunication Loop for update on the Webserver."
        n49 = Unbundle By Name(w152) -> ("WebServ"=w151:refnum<queue>, "UI"=w147:refnum<queue>)
        n50 = call-poly "EnqueueMessage.vi"("error in (no error)"=w156, "Message Data"=w154, "Message"="CurrentSRs", "Message Queue"=w147) -> ("error out"=w149:errorcluster)  [unwired: 6 in, 1 out]
        n51 = call-poly "EnqueueMessage.vi"("error in (no error)"=w149, "Message Data"=w154, "Message"="SetSRs", "Message Queue"=w151) -> ("error out"=w148:errorcluster)  [unwired: 6 in, 1 out]
        n52 = Get Date/Time In Seconds() -> (seconds since 1Jan1904=w145:timestamp)
        n53 = call-poly "EnqueueMessage.vi"("error in (no error)"=w148, "Message Data"=w145, "Message"="Last Update SRs", "Message Queue"=w147) -> ("error out"=w150:errorcluster)  [unwired: 6 in, 1 out]
      }
      frame "Log" {
        # "Forwards Log-Messages to the Log-Loop"
        n54 = Unbundle By Name(w158) -> ("Log"=w157:refnum<queue>)
        n55 = call-poly "EnqueueMessage.vi"("error in (no error)"=w162, "Message Data"=w159, "Message"=w160, "Message Queue"=w157) -> ("error out"=w161:errorcluster)  [unwired: 6 in, 1 out]
      }
      frame "TestClient" {
        # "Launches Test Client in Dialog-Loop"
        n56 = Unbundle By Name(w164) -> ("Dialog"=w163:refnum<queue>)
        n57 = call-poly "EnqueueMessage.vi"("error in (no error)"=w168, "Message Data"=w165, "Message"=w166, "Message Queue"=w163) -> ("error out"=w167:errorcluster)  [unwired: 6 in, 1 out]
      }
      frame "Settings" {
        # "Launch Settings Dialog to update INI-Global and File"
        n58 = Unbundle By Name(w172) -> ("Dialog"=w171:refnum<queue>)
        n59 = call-poly "EnqueueMessage.vi"("error in (no error)"=w174, "Message Data"=w169, "Message"=w170, "Message Queue"=w171) -> ("error out"=w173:errorcluster)  [unwired: 6 in, 1 out]
      }
      frame "UpdateSettings" {
        # "Write new settings to all queues"
        n60 = call "SendToAll.vi"("Priority Message? (F)"=TRUE, "error in (no error)"=w180, "Data"=w176, "Message"=w177, "Message Queues in"=w178) -> ("error out"=w179:errorcluster)  [unwired: 6 in]
      }
      frame "Error" {
        # "Error received from Errorhandler -> forward to Error Loop"
        n61 = Unbundle By Name(w184) -> ("Error"=w183:refnum<queue>)
        n62 = call-poly "EnqueueMessage.vi"("error in (no error)"=w186, "Message Data"=w181, "Message"=w182, "Message Queue"=w183) -> ("error out"=w185:errorcluster)  [unwired: 6 in, 1 out]
      }
      frame "Exit" {
        # "Forward exit-message to all loops, set Stop Global Variable \"true\" and stop MHL."
        n63 = call "SendToAll.vi"("Priority Message? (F)"=TRUE, "error in (no error)"=w192, "Data"=w187, "Message"=w189, "Message Queues in"=w191) -> ("error out"=w190:errorcluster)  [unwired: 6 in]
      }
      frame Default {
        # "Invalid message"
        n64 = xnode "Error Ring"("parameter 0"=w196) -> ("error out"=w197:errorcluster)
        n65 = Merge Errors(w197, w194) -> (w195:errorcluster)
      }
    }
    n66 = call "ErrorHandler.vi"("error in (no error)"=w113) -> ("error out"=w110:errorcluster)  [unwired: 10 in]
    n67 = Or(x=w110, y=w120) -> (x .or. y?=w111:bool)
  }
  n68 = call "ErrorLoop.vi"("Error In"=w12, "Message Queues"=w11) -> ("Error Out"=w17:errorcluster)  [unwired: 9 in]
  n69 = call "LoggingLoop.vi"("Error In"=w12, "Message Queues"=w11) -> ("Error Out"=w14:errorcluster)  [unwired: 9 in]
  n70 = call "TimingLoop.vi"("Error In"=w12, "Message Queues"=w11) -> ("Error Out"=w13:errorcluster)  [unwired: 9 in]
  n71 = call "DialogLoop.vi"("Error In"=w12, "Message Queues"=w11) -> ("Error Out"=w10:errorcluster)  [unwired: 9 in]
  n72 = call "WebServiceLoop.vi"("Error In"=w12, "Message Queues"=w11) -> ("Error Out"=w9:errorcluster)  [unwired: 9 in]
  n73 = call "OracleLoop.vi"("Error In"=w12, "Message Queues"=w11) -> ("Error Out"=w8:errorcluster)  [unwired: 9 in]
  n74 = Merge Errors(w15, w18, w20, w21, w17, w14, w13, w10, w9) -> (w1:errorcluster)
  n75 = call "OracleBusy.vi"("Mode"=enum16{"Busy", "Unbusy"}."Busy", "Error In"=w1) -> ("Error Out"=w6:errorcluster)  [unwired: 9 in]
  n76 = Merge Errors(w6, w8) -> (w7:errorcluster)
  n77 = call "OracleBusy.vi"("Mode"=enum16{"Busy", "Unbusy"}."Unbusy", "Error In"=w7) -> ("Error Out"=w3:errorcluster)  [unwired: 9 in]
  n78 = call "DestroyCommunication.vi"("error in (no error)"=w3, "Message Queues out"=w11) -> ("error out"=w2:errorcluster)  [unwired: 9 in]
  n79 = call <vilib>:"Simple Error Handler.vi"("error in (no error)"=w2) -> ("error out"=w16:errorcluster)  [unwired: 4 in, 4 out]
  n80 = disable-structure shown="RUN_TIME_ENGINE==True" {
    disable-tunnel: w16 -> [_ _]
    frame condition #0 (active) {
    }
    frame condition #1 {
      # "Call Quit LabVIEW if running as a built application."
      n81 = Quit LabVIEW() -> ()  [unwired: 1 in]
    }
  }
